vi "Record Nested Actor.vi"(8 "error in (no error)":errorcluster, 10 "Nested Mediated Asynchronous Actor's Message Transport":refnum<class "Message Transport Interface.lvclass">, 11 "Mediated Asynchronous Actor in":refnum<class "Mediated Asynchronous Actor.lvclass">) -> (0 "error out":errorcluster, 3 "Mediated Asynchronous Actor out":refnum<class "Mediated Asynchronous Actor.lvclass">)   [LabVIEW 2016, in "Stream Mediator.lvlib" / "Mediated Asynchronous Actor.lvclass"]
doc: "--\nCopyright © 2017 Composed SystemsI All rights reserved.\n\nAuthor: Jon McBee <jon.mcbee@composed.io>\n\nThis library is provided \"AS IS\" ,WITHOUT WARRANTIES OR\nCONDITIONS OF ANY KIND, either express or implied.\n\nComposed Systems -- composed.io\n\nStream 0.0.1.1\nJon McBee - Composed Systems\nCopyright (c) 2017, Composed Systems"
uses:
  <userlib>/Composed Systems/Stream/Mediator/Classes/Mediated Asynchronous Actor/Mediated Asynchronous Actor.lvclass
  <userlib>/Composed Systems/Stream/Mediator/Classes/Message Transport Interface/Message Transport Interface.lvclass
  <userlib>/Composed Systems/Stream/Mediator/Classes/Mediated Asynchronous Actor/Mediated Asynchronous Actor.lvclass/Mediated Asynchronous Actor.ctl
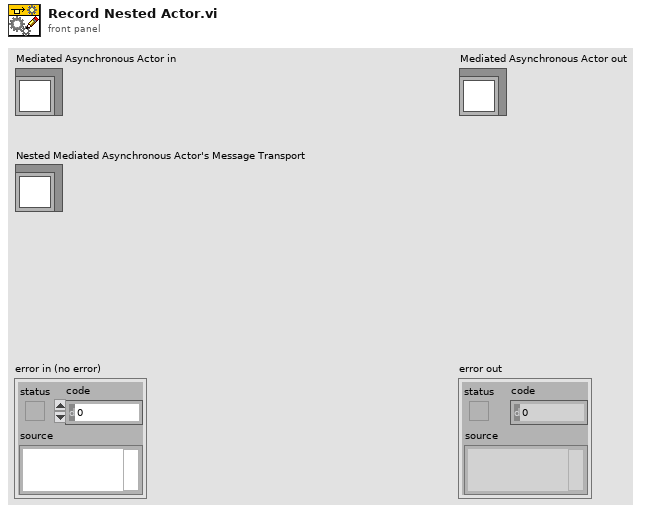
[diagram p1: front panel]
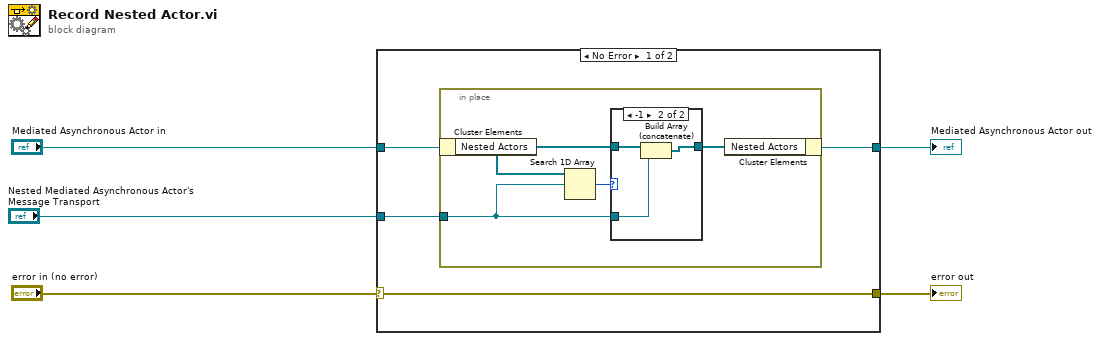
[diagram p0: block diagram]
diagram:
  n1 = case shown="No Error" "error in (no error)" {
    selector: "error in (no error)" -> [w9 w19]
    tunnel: [w9 w19] -> w1
    tunnel: [w6 w18] -> w4
    tunnel: "Mediated Asynchronous Actor in" -> [w8 w18]
    tunnel: "Nested Mediated Asynchronous Actor's Message Transport" -> [w7 _]
    frame No Error {
      n2 = in-place {
        in-place-border: w7 -> [w11]
        n3 = in-place-cluster #1(w8) -> ("Nested Actors"=w12:refnum<class "Message Transport Interface.lvclass">[])
        n4 = Search 1D Array(1D array=w12, element=w11) -> (index of element=w13:i32)  [unwired: 1 in]
        n5 = case shown="-1" w13 {
          tunnel: w12 -> [w14 w17]
          tunnel: w11 -> [_ w16]
          tunnel: [w14 w15] -> w10
          frame Default {
          }
          frame -1 {
            n6 = Build Array (concatenate)(w17, w16) -> (w15:refnum<class "Message Transport Interface.lvclass">[])
          }
        }
        n7 = in-place-cluster #1("Nested Actors"=w10) -> (w6:refnum<class "Mediated Asynchronous Actor.lvclass">)
      }
    }
    frame Error {
    }
  }
  "error out" <- w1
  "Mediated Asynchronous Actor out" <- w4
